vi "ExSubSave1Tif.vi"(2 "error in (no error)":errorcluster, 3 "File name":string, 4 "Image Handle":u32) -> (0 "error out":errorcluster, 1 "Image handle":u32)   [LabVIEW 2010]
panel:
  # "ExSubSave1Tif.vi : this sub-vi saves one\nimage to a tif file."
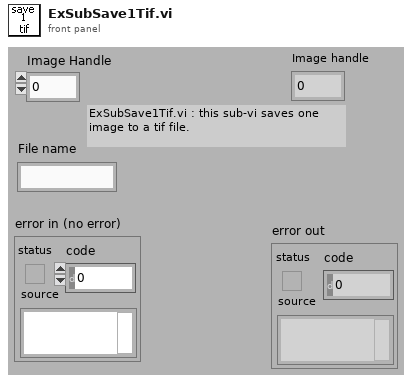
[diagram p1: front panel]
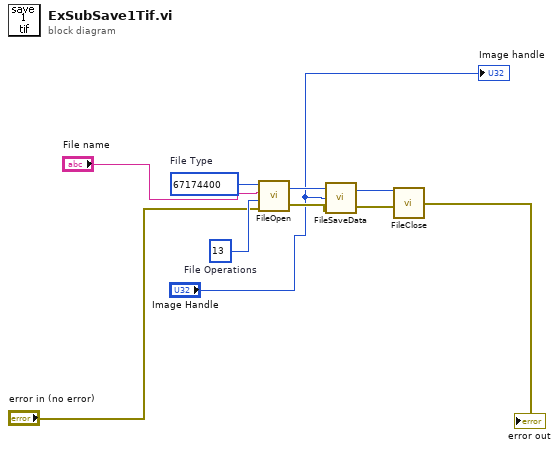
[diagram p0: block diagram]
diagram:
  w9 = 13  # File Operations
  w10 = 67174400  # File Type
  n1 = call <userlib>:"FileOpen.vi"("error in"="error in (no error)", "File Operations"=w9, "FileName"="File name", "File Type"=w10) -> ("error out"=w8:errorcluster, "File Handle"=w7:u32)
  n2 = call <userlib>:"FileSaveData.vi"("error in"=w8, "Image Handle"="Image Handle", "File Handle"=w7) -> ("error out"=w6:errorcluster, "File Handle"=w5:u32)
  n3 = call <userlib>:"FileClose.vi"("error in"=w6, "File Handle"=w5) -> ("error out"=→"error out":errorcluster)
  "Image handle" <- "Image Handle"
